vi "Read Defaults File.vi"(3 "Filename":string="TstDefts.txt") -> (0 "DirPath3":path=path "C:/This is dir #3", 1 "DirPath2":path=path "C:/This is dir #2", 2 "DirPath1":path=path "C:/This is dir #1", 4 "MiscPath10":path=path "C:/This is picture #10", 5 "MiscPath9":path=path "C:/This is picture #9", 6 "MiscPath8":path=path "C:/This is picture #8", 7 "MiscPath7":path=path "C:/This is picture #7", 8 "DirPath4":path=path "C:/This is dir #4", 9 "MiscPath6":path=path "C:/This is picture #6", 10 "DirPath5":path=path "C:/This is dir #5", 11 "MiscPath5":path=path "C:/This is picture #5", 12 "String1":string="Filename #1", 13 "MiscPath4":path=path "C:/This is picture #4", 14 "String2":string="Filename #2", 15 "MiscPath3":path=path "C:/This is picture #3", 16 "String3":string="Filename #3", 17 "MiscPath2":path=path "C:/This is picture #2", 18 "String4":string="Filename #4", 19 "MiscPath1":path=path "C:/This is picture #1", 20 "String5":string="Filename #5", 21 "BooleanArray":bool[](array[boolean])=[FALSE, TRUE, FALSE, TRUE, TRUE, FALSE], 22 "IntegerArray1":i32[](array[numeric])=[1, 2, 3, 4], 23 "ErrOut":bool, 24 "IntegerArray2":i32[](array[numeric])=[10, 20, 30, 40, 50], 25 "RealArray1":dbl[](array[numeric])=[1.1, 1.2, 1.3, 1.4] format="%.2f", 26 "RealArray2":dbl[](array[numeric])=[10.1, 20.2, 30.3, 40.4, 50.5] format="%.2f", 27 "StringArray":string[](array[string])=["String1", "String2", "String3"])   [LabVIEW 2013]
doc: "This vi reads a defaults ASCII file and decodes it into various paths, filenames, and arrays of strings, Booleans, integers and reals. An associated Write Defaults File.vi is required to create or update the defaults file. These vi's are very general and require external code to parse and build the arrays. All front-panel variables are read even if they are not used ( the arrays can be of any length ); the write vi creates placeholders automatically for unused items.\n\nModified to fit a standard VGA screen 6/1999 - MF Derr, AutoCon"
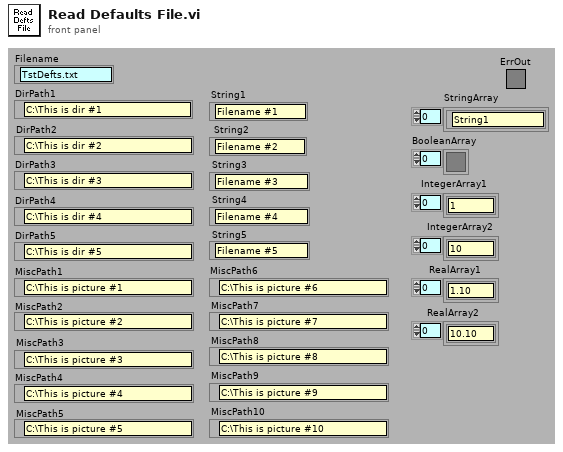
[diagram p1: front panel]
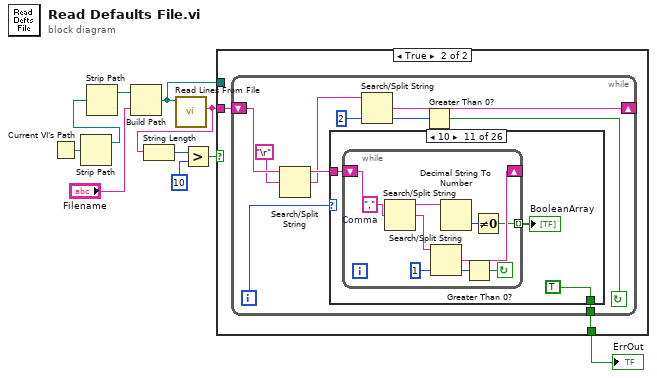
[diagram p0: block diagram]
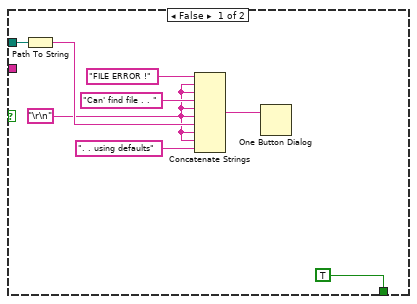
[diagram p2: hidden frame]
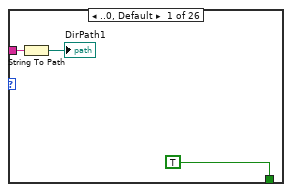
[diagram p3: hidden frame]
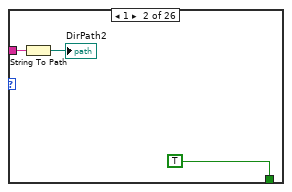
[diagram p4: hidden frame]
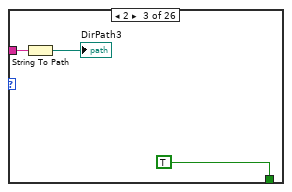
[diagram p5: hidden frame]
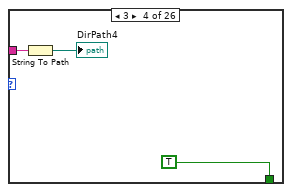
[diagram p6: hidden frame]
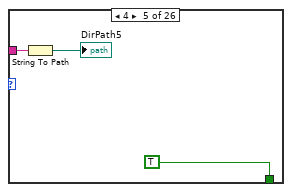
[diagram p7: hidden frame]
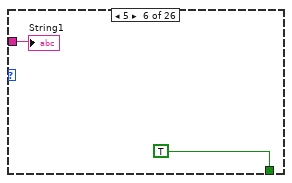
[diagram p8: hidden frame]
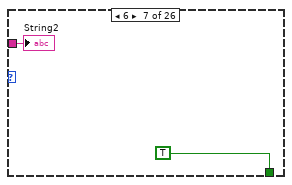
[diagram p9: hidden frame]
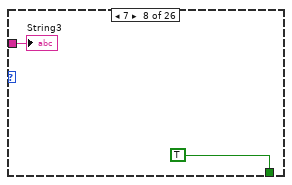
[diagram p10: hidden frame]
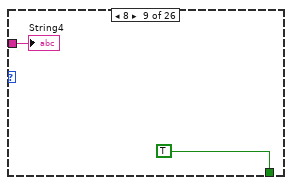
[diagram p11: hidden frame]
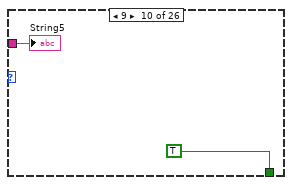
[diagram p12: hidden frame]
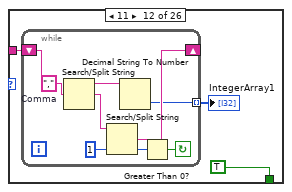
[diagram p13: hidden frame]
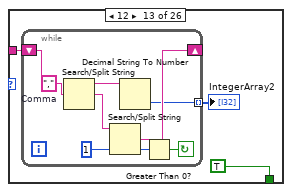
[diagram p14: hidden frame]
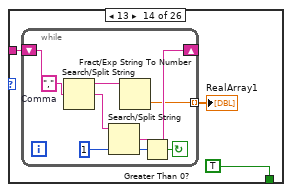
[diagram p15: hidden frame]
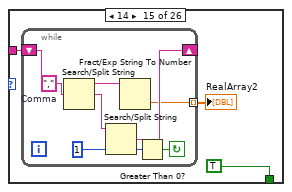
[diagram p16: hidden frame]
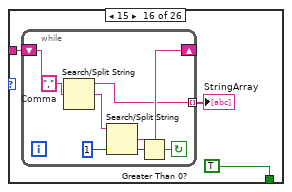
[diagram p17: hidden frame]
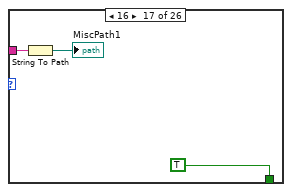
[diagram p18: hidden frame]
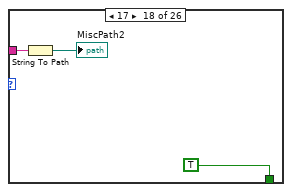
[diagram p19: hidden frame]
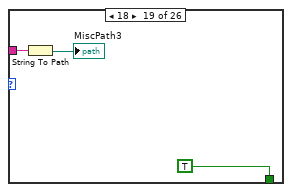
[diagram p20: hidden frame]
diagram:
  n1 = Current VI's Path() -> (path=w10:path)
  n2 = Strip Path(path=w10) -> (stripped path=w9:path)  [unwired: 1 out]
  n3 = Strip Path(path=w9) -> (stripped path=w8:path)  [unwired: 1 out]
  n4 = Build Path(base path=w8, name or relative path="Filename") -> (appended path=w2:path)
  n5 = call <vilib>:"Read Lines From File.vi"("file path (dialog if empty)"=w2) -> ("line string"=w6:string)  [unwired: 5 in, 3 out]
  n6 = String Length(string=w6) -> (length=w5:i32)
  n7 = Greater?(x=w5, y=10) -> (0:w3:bool)
  n8 = case shown="True" w3 {
    tunnel: w6 -> [_ w20]
    tunnel: w2 -> [w18 _]
    tunnel: [TRUE w19] -> w1
    frame False {
      w13 = "\r\n"
      n9 = Path To String(path=w18) -> (string=w14:string)
      n10 = Concatenate Strings("FILE ERROR !", w13, w13, "Can' find file . . ", w13, w13, w14, w13, w13, ". . using defaults") -> (w16:string)
      n11 = One Button Dialog(message=w16) -> ()  [unwired: 1 in, 1 out]
    }
    frame True {
      n12 = while {
        tunnel: [w22] -> w19
        shift-left: w20 -> [w30]
        shift-right: [w29] -> _
        i -> [w27]
        stop <- w25 continue-if-true
        n13 = Search/Split String(string=w30, search string/char (-)="\r") -> (substring before match=w24:string, match + rest of string=w23:string)  [unwired: 1 in, 1 out]
        n14 = case shown="10" w27 {
          tunnel: w24 -> [w33 w36 w39 w42 w45 w47 w48 w50 w52 w55 w57 w70 w82 w94 w106 w118 w130 w133 w136 w139 w142 w145 w148 w151 w154 w157]
          tunnel: [TRUE TRUE TRUE TRUE TRUE TRUE TRUE TRUE TRUE TRUE TRUE TRUE TRUE TRUE TRUE TRUE TRUE TRUE TRUE TRUE TRUE TRUE TRUE TRUE TRUE FALSE] -> w22
          frame ..0, Default {
            n15 = String To Path(string=w33) -> (path=→"DirPath1":path)
          }
          frame 1 {
            n16 = String To Path(string=w36) -> (path=→"DirPath2":path)
          }
          frame 2 {
            n17 = String To Path(string=w39) -> (path=→"DirPath3":path)
          }
          frame 3 {
            n18 = String To Path(string=w42) -> (path=→"DirPath4":path)
          }
          frame 4 {
            n19 = String To Path(string=w45) -> (path=→"DirPath5":path)
          }
          frame 5 {
            "String1" <- w47
          }
          frame 6 {
            "String2" <- w48
          }
          frame 7 {
            "String3" <- w50
          }
          frame 8 {
            "String4" <- w52
          }
          frame 9 {
            "String5" <- w55
          }
          frame 10 {
            n20 = while {
              tunnel: [w59] -> w56 mode=indexing
              shift-left: w57 -> [w67]
              shift-right: [w60] -> _
              stop <- w62 continue-if-true
              w68 = ","  # Comma
              n21 = Search/Split String(string=w67, search string/char (-)=w68) -> (substring before match=w65:string, match + rest of string=w61:string)  [unwired: 1 in, 1 out]
              n22 = Search/Split String(string=w61, offset (0)=1) -> (match + rest of string=w60:string, offset of match=w63:i32)  [unwired: 1 in, 1 out]
              n23 = Decimal String To Number(string=w65) -> (number=w66:i32)  [unwired: 2 in, 1 out]
              n24 = Greater Than 0?(x=w63) -> (x > 0?=w62:bool)
              n25 = Not Equal To 0?(x=w66) -> (x != 0?=w59:bool)
            }
            "BooleanArray" <- w56
          }
          frame 11 {
            n26 = while {
              tunnel: [w72] -> w69 mode=indexing
              shift-left: w70 -> [w79]
              shift-right: [w73] -> _
              stop <- w75 continue-if-true
              w80 = ","  # Comma
              n27 = Search/Split String(string=w79, search string/char (-)=w80) -> (substring before match=w78:string, match + rest of string=w74:string)  [unwired: 1 in, 1 out]
              n28 = Search/Split String(string=w74, offset (0)=1) -> (match + rest of string=w73:string, offset of match=w76:i32)  [unwired: 1 in, 1 out]
              n29 = Decimal String To Number(string=w78) -> (number=w72:i32)  [unwired: 2 in, 1 out]
              n30 = Greater Than 0?(x=w76) -> (x > 0?=w75:bool)
            }
            "IntegerArray1" <- w69
          }
          frame 12 {
            n31 = while {
              tunnel: [w84] -> w81 mode=indexing
              shift-left: w82 -> [w91]
              shift-right: [w85] -> _
              stop <- w87 continue-if-true
              w92 = ","  # Comma
              n32 = Search/Split String(string=w91, search string/char (-)=w92) -> (substring before match=w90:string, match + rest of string=w86:string)  [unwired: 1 in, 1 out]
              n33 = Search/Split String(string=w86, offset (0)=1) -> (match + rest of string=w85:string, offset of match=w88:i32)  [unwired: 1 in, 1 out]
              n34 = Decimal String To Number(string=w90) -> (number=w84:i32)  [unwired: 2 in, 1 out]
              n35 = Greater Than 0?(x=w88) -> (x > 0?=w87:bool)
            }
            "IntegerArray2" <- w81
          }
          frame 13 {
            n36 = while {
              tunnel: [w96] -> w93 mode=indexing
              shift-left: w94 -> [w103]
              shift-right: [w97] -> _
              stop <- w99 continue-if-true
              w104 = ","  # Comma
              n37 = Search/Split String(string=w103, search string/char (-)=w104) -> (substring before match=w102:string, match + rest of string=w98:string)  [unwired: 1 in, 1 out]
              n38 = Search/Split String(string=w98, offset (0)=1) -> (match + rest of string=w97:string, offset of match=w100:i32)  [unwired: 1 in, 1 out]
              n39 = Fract/Exp String To Number(string=w102) -> (number=w96:dbl)  [unwired: 3 in, 1 out]
              n40 = Greater Than 0?(x=w100) -> (x > 0?=w99:bool)
            }
            "RealArray1" <- w93
          }
          frame 14 {
            n41 = while {
              tunnel: [w108] -> w105 mode=indexing
              shift-left: w106 -> [w115]
              shift-right: [w109] -> _
              stop <- w111 continue-if-true
              w116 = ","  # Comma
              n42 = Search/Split String(string=w115, search string/char (-)=w116) -> (substring before match=w114:string, match + rest of string=w110:string)  [unwired: 1 in, 1 out]
              n43 = Search/Split String(string=w110, offset (0)=1) -> (match + rest of string=w109:string, offset of match=w112:i32)  [unwired: 1 in, 1 out]
              n44 = Fract/Exp String To Number(string=w114) -> (number=w108:dbl)  [unwired: 3 in, 1 out]
              n45 = Greater Than 0?(x=w112) -> (x > 0?=w111:bool)
            }
            "RealArray2" <- w105
          }
          frame 15 {
            n46 = while {
              tunnel: [w120] -> w117 mode=indexing
              shift-left: w118 -> [w126]
              shift-right: [w121] -> _
              stop <- w123 continue-if-true
              w127 = ","  # Comma
              n47 = Search/Split String(string=w126, search string/char (-)=w127) -> (substring before match=w120:string, match + rest of string=w122:string)  [unwired: 1 in, 1 out]
              n48 = Search/Split String(string=w122, offset (0)=1) -> (match + rest of string=w121:string, offset of match=w124:i32)  [unwired: 1 in, 1 out]
              n49 = Greater Than 0?(x=w124) -> (x > 0?=w123:bool)
            }
            "StringArray" <- w117
          }
          frame 16 {
            n50 = String To Path(string=w130) -> (path=→"MiscPath1":path)
          }
          frame 17 {
            n51 = String To Path(string=w133) -> (path=→"MiscPath2":path)
          }
          frame 18 {
            n52 = String To Path(string=w136) -> (path=→"MiscPath3":path)
          }
          frame 19 {
            n53 = String To Path(string=w139) -> (path=→"MiscPath4":path)
          }
          frame 20 {
            n54 = String To Path(string=w142) -> (path=→"MiscPath5":path)
          }
          frame 21 {
            n55 = String To Path(string=w145) -> (path=→"MiscPath6":path)
          }
          frame 22 {
            n56 = String To Path(string=w148) -> (path=→"MiscPath7":path)
          }
          frame 23 {
            n57 = String To Path(string=w151) -> (path=→"MiscPath8":path)
          }
          frame 24 {
            n58 = String To Path(string=w154) -> (path=→"MiscPath9":path)
          }
          frame 25 {
            n59 = String To Path(string=w157) -> (path=→"MiscPath10":path)
          }
        }
        n60 = Search/Split String(string=w23, offset (0)=2) -> (match + rest of string=w29:string, offset of match=w26:i32)  [unwired: 1 in, 1 out]
        n61 = Greater Than 0?(x=w26) -> (x > 0?=w25:bool)
      }
    }
  }
  "ErrOut" <- w1
